vi "Controller_2_2_Proportional.vi"() -> ()   [LabVIEW 2019]
uses:
  <vilib>/myRIO/Instrument Drivers/Onboard IO/AI/typedefs/AI Reference.ctl
  <vilib>/myRIO/Common/Instrument Driver Framework/Utilities/typedefs/myRIO Generic Hardware Reference.ctl
  <vilib>/myRIO/Common/Instrument Driver Framework/Utilities/typedefs/Hardware Version Enum.ctl
  <vilib>/myRIO/Common/Instrument Driver Framework/Utilities/typedefs/myRIO v1.0 Reference.ctl
  <vilib>/myRIO/Common/Instrument Driver Framework/Utilities/typedefs/Generic FPGA Reference.ctl
  <vilib>/myRIO/Common/Instrument Driver Framework/myRIO v1.0/AI/typedefs/AI Channels List.ctl
  <vilib>/myRIO/Common/Instrument Driver Framework/myRIO v1.0/AI/typedefs/AI Channels Enum.ctl
  <vilib>/myRIO/Common/Instrument Driver Framework/Utilities/typedefs/Analog Scaling Constants List.ctl
  <vilib>/myRIO/Common/Instrument Driver Framework/Utilities/typedefs/Analog Scaling Constants.ctl
  <vilib>/userDefined/High Color/nirio_resource_hc.ctl
  <vilib>/Simulation/Scripting/Companion Diagram/SimConfigNode/SimParams.ctl
  <vilib>/Simulation/Scripting/Companion Diagram/SimConfigNode/_simSolvers.ctl
  <vilib>/Simulation/Implementation/Shared/SIMSCR Execution Mode.ctl
  <vilib>/Simulation/Param Hierarchy/Typedefs/SIMPH Param Control Actions.ctl
  <vilib>/myRIO/Instrument Drivers/Onboard IO/PWM/typedefs/PWM Reference.ctl
  <vilib>/myRIO/Common/Instrument Driver Framework/myRIO v1.0/PWM/typedefs/PWM Channels Enum.ctl
  <vilib>/myRIO/Instrument Drivers/Onboard IO/PWM/typedefs/PWM Configuration.ctl
  <vilib>/myRIO/Common/Instrument Driver Framework/Utilities/vis/Is FPGA Ref Available.vi
  <vilib>/myRIO/Common/Instrument Driver Framework/myRIO v1.0/AI/vis/myRIO v1.1 Open AI.vi
  <vilib>/myRIO/Instrument Drivers/Onboard IO/AI/vis/Read.vi
  <vilib>/Simulation/Implementation/Shared/NILVSim_ParamChanged.vi
  <vilib>/Simulation/Implementation/Shared/NILVSIM_BeginStep.vi
  <vilib>/Simulation/Implementation/Shared/NILVSim_Manager.vi
  <vilib>/Utility/error.llb/Clear Errors.vi
  <vilib>/Simulation/Implementation/Shared/NILVSim_FinalizeModel.vi
  <vilib>/myRIO/Common/Instrument Driver Framework/myRIO v1.0/PWM/vis/myRIO v1.1 Open PWM.vi
  <vilib>/myRIO/Instrument Drivers/Onboard IO/PWM/vis/Set Duty Cycle and Frequency.vi
  <vilib>/myRIO/Common/Instrument Driver Framework/Utilities/vis/Validate Channels.vi
  <vilib>/myRIO/Common/Instrument Driver Framework/myRIO v1.0/AI/vis/myRIO v1.0 Reserve AI.vi
  <vilib>/myRIO/Common/Instrument Driver Framework/myRIO v1.0/PWM/vis/myRIO v1.0 Reserve PWM.vi
  <vilib>/myRIO/Common/Instrument Driver Framework/myRIO v1.0/UART/vis/myRIO v1.0 Close UART.vi
  <vilib>/myRIO/Common/Instrument Driver Framework/myRIO v1.0/AI/vis/myRIO v1.0 Build MUX Configuration AI.vi
  <vilib>/myRIO/Common/Instrument Driver Framework/myRIO v1.0/Resource Manager/vis/myRIO v1.0 Reserve Channel List.vi
  <vilib>/myRIO/Common/Instrument Driver Framework/myRIO v1.0/PWM/vis/myRIO v1.0 Build MUX Configuration PWM.vi
  <vilib>/myRIO/Common/Instrument Driver Framework/myRIO v1.0/Resource Manager/vis/myRIO v1.0 Reserve Channel.vi
  <vilib>/myRIO/Common/Instrument Driver Framework/myRIO v1.0/Resource Manager/vis/myRIO v1.0 Unreserve Channel.vi
  <vilib>/myRIO/Common/Instrument Driver Framework/myRIO v1.0/Resource Manager/vis/myRIO v1.0 Create Configuration List.vi
  <vilib>/myRIO/Common/Instrument Driver Framework/myRIO v1.0/Resource Manager/vis/myRIO v1.0 Build Mutex Name.vi
  <vilib>/Utility/VariantDataType/GetNumericInfo.vi
  <vilib>/Utility/error.llb/Error Cluster From Error Code.vi
  <vilib>/myRIO/Common/Instrument Driver Framework/myRIO v1.0/myRIO v1.1 Open.vi
  <vilib>/myRIO/Common/Instrument Driver Framework/myRIO v1.0/AI/vis/myRIO v1.0 Get Scaling Constants AI.vi
  <vilib>/myRIO/Common/Instrument Driver Framework/Utilities/vis/IO Manager.vi
  <vilib>/myRIO/Common/Instrument Driver Framework/Utilities/vis/Configuration Manager.vi
  <vilib>/myRIO/Common/Instrument Driver Framework/myRIO v1.0/myRIO v1.0 Close.vi
  <vilib>/myRIO/Common/Instrument Driver Framework/myRIO v1.0/AI/vis/myRIO v1.0 Read AI.vi
  <vilib>/imath/engines/lvmath2/RunTimeEngine/Managers/WorkSpace/UID Generator.vi
  <vilib>/imath/engines/lvmath2/RunTimeEngine/RunTimeType/NIMS_RunTimeType_From StrictType (excl LVString).vi
  <instcachedir>/0/NIMS_RunTimeType_From StrictType (excl LVString)_D8AFBA86A94845AAA577C895450664BD.lvgen/NIMS_RunTimeType_From StrictType (excl LVString)_D8AFBA86A94845AAA577C895450664BD_000.vi
  <vilib>/imath/engines/lvmath2/RunTimeEngine/LocalVariableDefStatement/MC_LocalVariableDefStatement_Display.vi
  <vilib>/imath/engines/lvmath2/RunTimeEngine/Managers/SymbolTable/Clear UID.vi
  <vilib>/imath/engines/lvmath2/RunTimeEngine/NodeEndStatement/NIMS_NodeEndStatement_Output.vi
  <instcachedir>/0/NIMS_NodeEndStatement_Output_53EC0D466D134D7ABD903AC30B43404B.lvgen/NIMS_NodeEndStatement_Output_53EC0D466D134D7ABD903AC30B43404B_001.vi
  <vilib>/imath/engines/lvmath2/RunTimeEngine/ErrorHandling/NIMS_Finalize Error.vi
  <vilib>/Simulation/Implementation/Shared/SIM Unbundle Sim Info.vi
  <vilib>/Simulation/Implementation/Shared/NILVSim_Initialize.vi
  <vilib>/Simulation/Utility/Implementation/NILVSim Get Time and IsAcceptedStep.vi
  <vilib>/Simulation/Implementation/Shared/SIMSH Read Queue.vi
  <vilib>/Simulation/Implementation/Shared/NILVSim_GetModelError.vi
  <vilib>/Simulation/Implementation/Shared/SIM Bundle Sim Info.vi
  <vilib>/myRIO/Common/Instrument Driver Framework/myRIO v1.0/Resource Manager/vis/myRIO v1.0 Configure IO.vi
  <vilib>/myRIO/Common/Instrument Driver Framework/myRIO v1.0/PWM/vis/myRIO v1.0 Write PWM.vi
  <vilib>/addons/control/pid/pid.llb/PID (DBL).vi
  <vilib>/myRIO/Common/Instrument Driver Framework/Utilities/vis/FPGA Ref Manager.vi
  <vilib>/myRIO/Common/Instrument Driver Framework/myRIO v1.0/myRIO v1.0 Reset FPGA.vi
  <vilib>/myRIO/Common/Instrument Driver Framework/myRIO v1.0/IRQ/vis/myRIO v1.0 IRQ Info FGV.vi
  <vilib>/myRIO/Common/Instrument Driver Framework/myRIO v1.0/IRQ/vis/myRIO v1.0 Timer IRQ Info FGV.vi
  <vilib>/myRIO/Common/Instrument Driver Framework/myRIO v1.0/IRQ/vis/myRIO v1.0 ISR Agent.vi
  <vilib>/myRIO/Instrument Drivers/Utilities/vis/Reset Index.vi
  <vilib>/myRIO/Common/Instrument Driver Framework/myRIO v1.0/Resource Manager/vis/myRIO v1.0 Block Write Resource Manager.vi
  <vilib>/myRIO/Express VI/Onboard IO/AI/AI Express VI.xnode
  <vilib>/myRIO/Instrument Drivers/Onboard IO/AI/vis/myRIO AI Open.xnode
  <vilib>/Simulation/Implementation/XNodeFramework/SimXNode/SimX.xnode
  Subsystems/RateLimit.vi
  <vilib>/Simulation/Scripting/Companion Diagram/SimConfigNode/SimDog.xnode
  <vilib>/myRIO/Express VI/Onboard IO/PWM/PWM Express VI.xnode
  <vilib>/myRIO/Instrument Drivers/Onboard IO/PWM/vis/myRIO PWM Open.xnode
  <vilib>/myRIO/Instrument Drivers/Onboard IO/PWM/PWM.lvlib
  <vilib>/myRIO/Instrument Drivers/Onboard IO/AI/AI.lvlib
  <vilib>/imath/engines/lvmath2/RunTimeEngine/Managers/SymbolTable/NIMS_WorkSpace.lvlib
  <vilib>/addons/control/pid/NI_PID_pid.lvlib
  <vilib>/ptbypt/NI_PtbyPt.lvlib
  <vilib>/myRIO/Instrument Drivers/Utilities/Utilities.lvlib
  <vilib>/Simulation/Implementation/Shared/NI_SIM_Implementation.lvlib
panel:
  in  "emax 2":dbl
  in  "offset 2":dbl
  out "Duty Cycle 2":dynamicdata(graph)
  in  "emax":dbl
  in  "offset":dbl
  in  "Slew":dbl
  out "Deflate":dbl
  out "Inflate":dbl
  out "Deflate":bool
  out "Inflate":bool
  in  "deadband":dbl
  out "double precision float":dbl
  out "Arbitrary Signal":dynamicdata(graph)
  out "Duty Cycle":dynamicdata(graph)
  out "Pressure Actuator":dynamicdata(graph)
  out "Pressures Actuator":cluster{dbl, dbl}(knob)={0.0, 8.870406975580165} scale=0.0..120.0
  in  "stop":bool
  out "VA_sensor":dbl format="%#.3g"
  out "Pressures Receiver":cluster{dbl, dbl}(knob)={0.0, 8.870406975580165} scale=0.0..120.0
  in  "Setpoint Preceiver":dbl(slide) scale=0.0..100.0
  out "V_Rsensor":dbl format="%#.3g"
  in  "PID Motor":T1={"proportional gain (Kc)"=0.01, "integral time (Ti, min)"=0.005, "derivative time (Td, min)"=0.0} {"derivative time (Td, min)" format="%.3f"; "integral time (Ti, min)" format="%.3f"; "proportional gain (Kc)" format="%.3f"}
  out "Duty cycle Motor":dbl(knob) scale=0.0..1.0
  in  "milliseconds to wait":u32=100
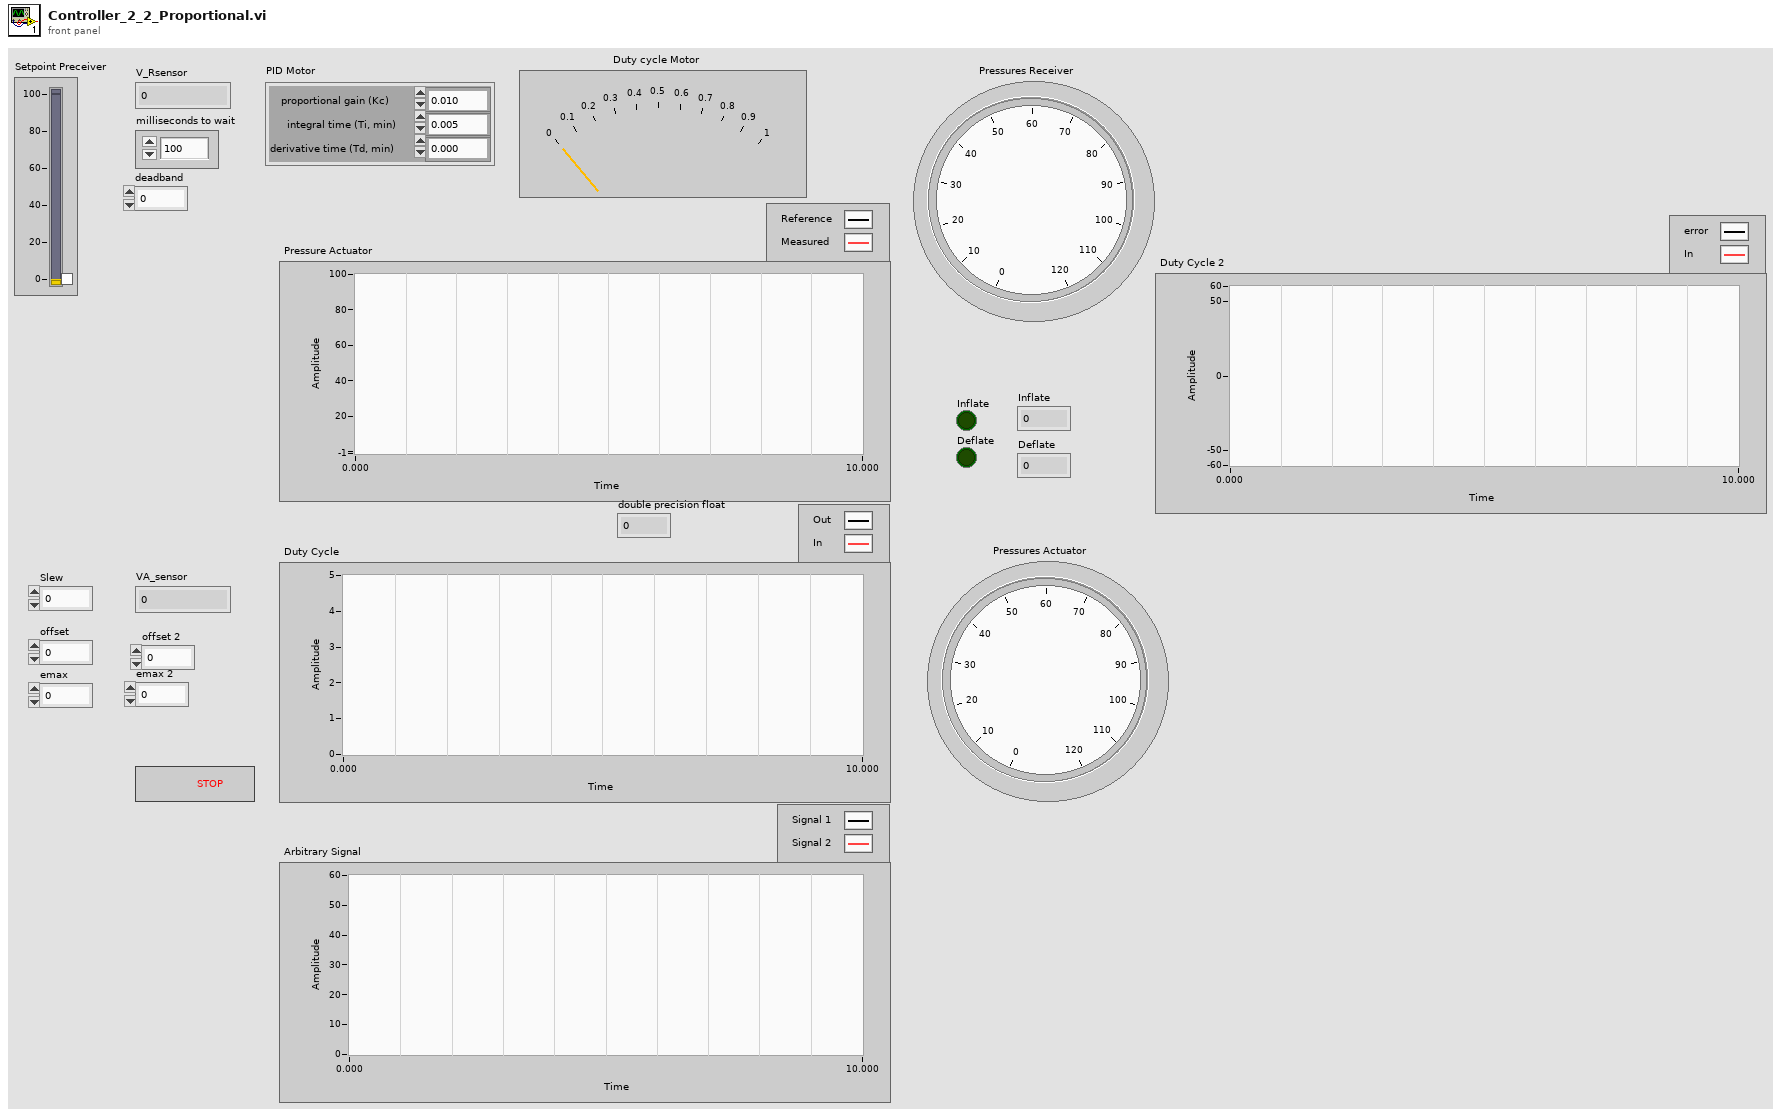
[diagram p1: front panel]
types:
  T1 = cluster{"proportional gain (Kc)":dbl, "integral time (Ti, min)":dbl, "derivative time (Td, min)":dbl}
  T2 = enum16{"Simulate to Completion", "Single Time-Step Simulation (Fixed Step Only)"}
  T3 = typedef "SIMSCR Execution Mode.ctl" = enum16{"Simulate to Completion", "Single Time-Step Simulation (Fixed Step Only)"}
  T4 = typedef "SIMPH Param Control Actions.ctl" = enum16{"get params", "set params"}
  T5 = cluster{"SIMSH Sim Time":dbl, "Negate":cluster{"-x":dbl}, "input":dbl, "Rate Limiter":cluster{"output":dbl}}
  T6 = typedef "SimParams.ctl" = cluster{"Initial Time (s)":dbl, "Final Time (s)":dbl, "Step Size (s)":dbl, "ODE Solver":T7, "Minimum Step Size (s)":dbl, "Maximum Step Size (s)":dbl, "Relative Tolerance":dbl, "Absolute Tolerance":dbl, "Software Timing":bool, "Initial Step Size (s)":dbl, "Automatic Fixed Step Size?":bool, "Automatic Discrete Step Size?":bool, "Discrete Step Size (s)":dbl, "Calculate using Time Step":bool, "Solver Wired?":bool, "Prev.Frm.Expected End":u64, "Prev.Frm.Actual End":u64, "Prev.Frm.Finished Late?":bool, "Prev.Iter.Expected End":u64, "Prev.Iter.Actual End":u64, "Prev.Iter.Finished Late?":bool, "Expected Iteration Start":u64, "Actual Iteration Start":u64, "Expected Frame Start":u64, "Actual Frame Start":u64, "Source Name":string, "Name":string, "Period":i64, "Deadline":i64, "Offset":i64, "Start":i64, "Priority":i32, "Timeout":i32, "Processor":i32, "Mode":enum32{"No Change", "Process missed periods, maintain original phase", "Discard missed periods, maintain original phase", "Process missed periods, ignore original phase", "Discard missed periods, ignore original phase"}, "Wakeup reason":enum32{"Normal", "Aborted", "Asynchronous wakeup", "Timing source error", "Timed loop error", "Timeout"}, "Error":errorcluster, "Source Type":string, "Secondary Source Type":string, "Global End Time":u64, "Global Start Time":u64, "Full Solver Reset":bool, "Execution Mode":T3, "Nan/Inf Check":bool, "Custom Solver Library":string, "Solver Is Variable":bool, "custom solver name":string, "Signal Collection Decimation":u32}
  T7 = typedef "_simSolvers.ctl" = enum16{"Runge-Kutta 1 (Euler)", "Runge-Kutta 2", "Runge-Kutta 3", "Runge-Kutta 4", "Runge-Kutta 23 (variable)", "Runge-Kutta 45 (variable)", "BDF (variable)", "Adams-Moulton (variable)", "Rosenbrock (variable)", "Discrete States Only", "SDIRK 4 (variable)", "Radau 5 (variable)", "Radau 9 (variable)", "Radau 13 (variable)", "Radau [Variable Order] (variable)", "Gear's Method (variable)", "Linearizer", "State Query", "Trim Eval", "Custom Solver"}
  T8 = typedef "PWM.lvlib/PWM Reference.ctl" = cluster{"myRIO Reference":T9, "PWM Channels Enum":T13, "PWM Configuration":T14}
  T9 = typedef "myRIO Generic Hardware Reference.ctl" = cluster{"myRIO Model":T10, "myRIO Hardware Reference":T11}
  T10 = typedef "Hardware Version Enum.ctl" = enum16{"Unknown", "myRIO-1900", "myRIO-1950", "roboRIO", "NI ELVIS RIO CM", "ELVIS III"}
  T11 = typedef "myRIO v1.0 Reference.ctl" = cluster{"Generic FPGA Reference":T12, "Allow multiple opens":bool}
  T12 = typedef "Generic FPGA Reference.ctl" = refnum<k20>
  T13 = typedef "PWM Channels Enum.ctl" = enum16{"Not Connected", "C/PWM0", "C/PWM1", "A/PWM0", "A/PWM1", "A/PWM2", "A/PWM3", "A/PWM4", "A/PWM5", "A/PWM6", "A/PWM7", "A/PWM8", "A/PWM9", "A/PWM10", "A/PWM11", "A/PWM12", "A/PWM13", "A/PWM14", "A/PWM15", "A/PWM16", "A/PWM17", "A/PWM18", "A/PWM19", "B/PWM0", "B/PWM1", "B/PWM2", "B/PWM3", "B/PWM4", "B/PWM5", "B/PWM6", "B/PWM7", "B/PWM8", "B/PWM9", "B/PWM10", "B/PWM11", "B/PWM12", "B/PWM13", "B/PWM14", "B/PWM15", "B/PWM16", "B/PWM17", "B/PWM18", "B/PWM19", "PWM/PWM0", "PWM/PWM1", "PWM/PWM2", "PWM/PWM3", "PWM/PWM4", "PWM/PWM5", "PWM/PWM6", "PWM/PWM7", "PWM/PWM8", "PWM/PWM9"}
  T14 = typedef "PWM.lvlib/PWM Configuration.ctl" = cluster{"Frequency":dbl, "Duty Cycle":dbl}
  T15 = typedef "nirio_resource_hc.ctl" = tag
  T16 = typedef "AI.lvlib/AI Reference.ctl" = cluster{"myRIO Reference":T9, "AI Channels List":T17, "AI Scaling Constants List":T19}
  T17 = typedef "AI Channels List.ctl" = T18[]
  T18 = typedef "AI Channels Enum.ctl" = enum16{"Not Connected", "AudioIn/Left", "AudioIn/Right", "C/AI0", "C/AI1", "A/AI0", "A/AI1", "A/AI2", "A/AI3", "A/AI4", "A/AI5", "A/AI6", "A/AI7", "B/AI0", "B/AI1", "B/AI2", "B/AI3", "B/AI4", "B/AI5", "B/AI6", "B/AI7", "AI/AI0", "AI/AI1", "AI/AI2", "AI/AI3", "A/AI0 (DIFF)", "A/AI1 (DIFF)", "A/AI2 (DIFF)", "A/AI3 (DIFF)", "B/AI0 (DIFF)", "B/AI1 (DIFF)", "B/AI2 (DIFF)", "B/AI3 (DIFF)"}
  T19 = typedef "Analog Scaling Constants List.ctl" = T20[]
  T20 = typedef "Analog Scaling Constants.ctl" = cluster{"LSB Weight (Volts)":dbl, "Offset (Volts)":dbl, "Signed?":bool}
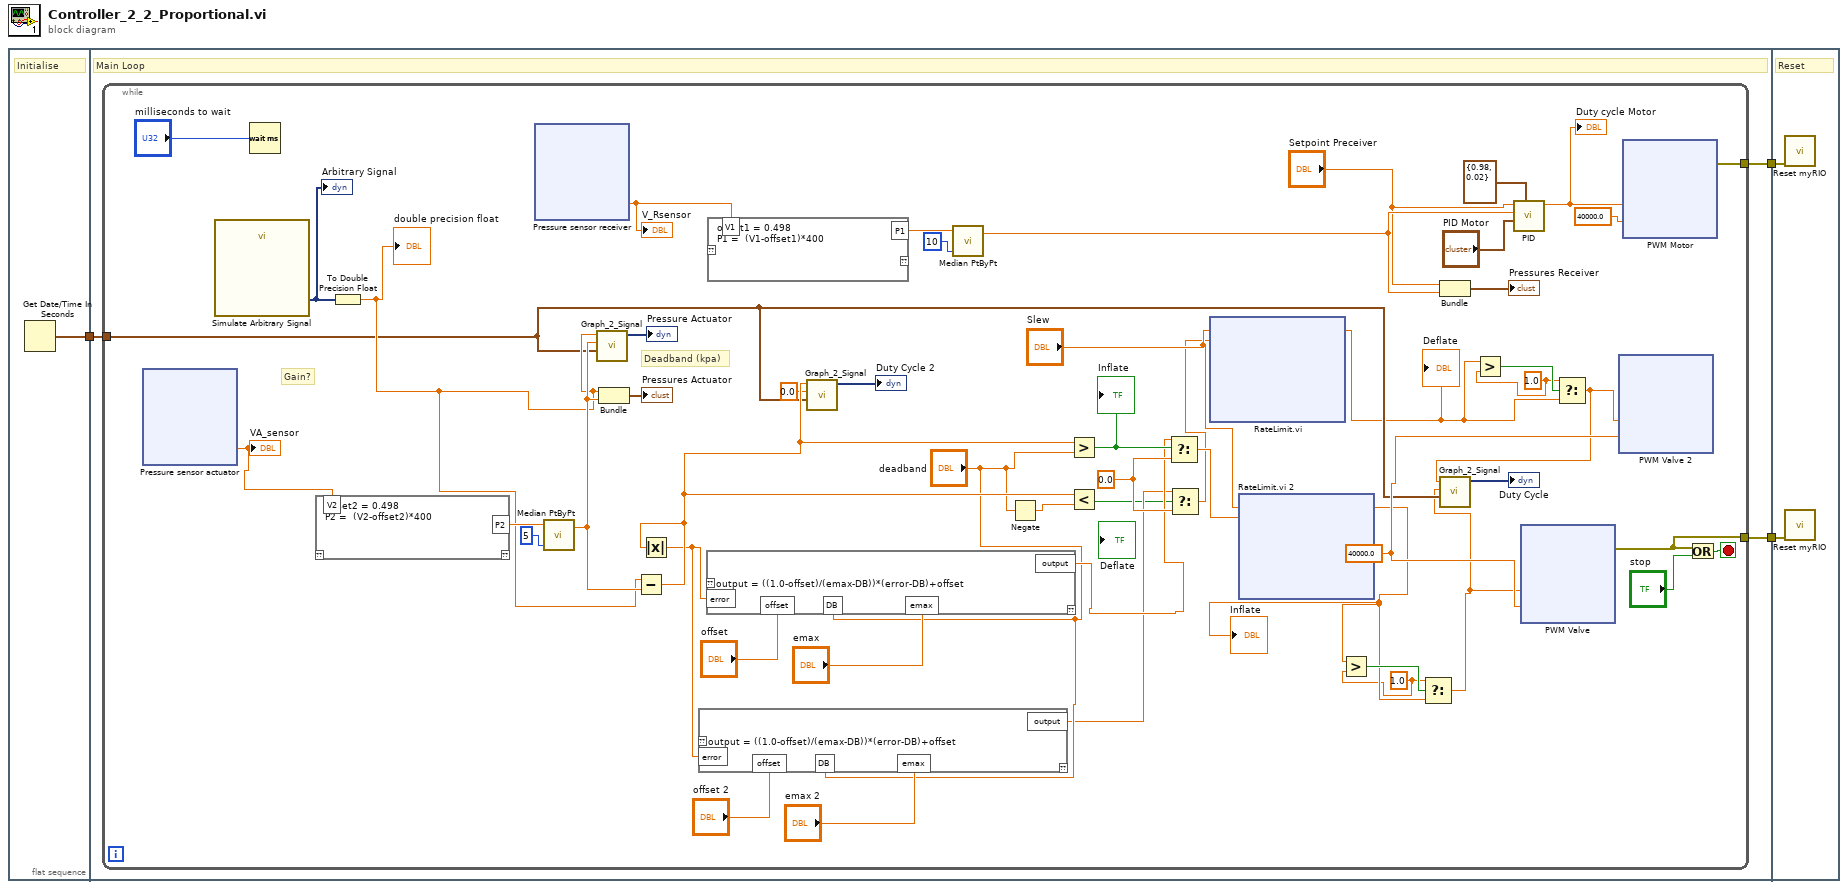
[diagram p0: block diagram]
diagram:
  n1 = flat-sequence {
    tunnel: [w4] -> w3
    tunnel: [w7] -> w2
    tunnel: [w6] -> w1
    tunnel: w3 -> [w5]
    tunnel: w2 -> [w938]
    tunnel: w1 -> [w937]
    frame #0 {
      # "Initialise"
      n2 = Get Date/Time In Seconds() -> (seconds since 1Jan1904=w4:timestamp)
    }
    frame #1 {
      # "Main Loop"
      n3 = while {
        tunnel: [w58] -> w7
        tunnel: [w47] -> w6
        tunnel: w5 -> [w23]
        stop <- w57 stop-if-true
        w11 = 1.0 ("t")
        w13 = 1.0 ("t")
        w34 = 0.0 ("f")
        w37 = 40000.0 ("Frequency [Hz]")
        # "Deadband (kpa)"
        # "Gain?"
        n4 = xnode "Pressure sensor actuator"() -> ("B/AI1 (Pin 5)"=w42:dbl)  [unwired: 1 in, 1 out]
        "VA_sensor" <- w42
        n5 = call "Simulate Arbitrary Signal"() -> ("Signal"=w40:dynamicdata)  [unwired: 9 in, 2 out]
        "Arbitrary Signal" <- w40
        n6 = Wait (ms)(milliseconds to wait="milliseconds to wait") -> ()  [unwired: 1 out]
        n7 = mathscript code="offset2 = 0.498\nP2 =  (V2-offset2)*400"("V2"=w42) -> ("P2"=w56:dbl)  [unwired: 1 in, 1 out]
        n8 = To Double Precision Float(number=w40) -> (double precision float=w27:dbl)
        "double precision float" <- w27
        n9 = xnode "Pressure sensor receiver"() -> ("B/AI0 (Pin 3)"=w41:dbl)  [unwired: 1 in, 1 out]
        "V_Rsensor" <- w41
        n10 = call <vilib>:"Median PtByPt.vi"("sample length"=5, "x"=w56) -> ("median"=w36:dbl)  [unwired: 2 in, 1 out]
        n11 = call "Graph_2_Signal.vi"("y"=w23, "Dynamic Data 2"=w36, "Dynamic Data 1"=w27) -> ("Signals"=→"Pressure Actuator":dynamicdata)  [unwired: 8 in]
        n12 = Bundle(w27, "median"=w36) -> (→"Pressures Actuator":cluster{dbl, "median":dbl})  [unwired: 1 in]
        n13 = Subtract(x=w27, y=w36) -> (x-y=w24:dbl)
        n14 = Absolute Value(x=w24) -> (abs(x)=w19:dbl)
        n15 = mathscript code="output = ((1.0-offset)/(emax-DB))*(error-DB)+offset"("error"=w19, "offset"="offset 2", "DB"="deadband", "emax"="emax 2") -> ("output"=w17:dbl)  [unwired: 1 in, 1 out]
        n16 = mathscript code="output = ((1.0-offset)/(emax-DB))*(error-DB)+offset"("error"=w19, "offset"="offset", "DB"="deadband", "emax"="emax") -> ("output"=w26:dbl)  [unwired: 1 in, 1 out]
        n17 = mathscript code="offset1 = 0.498\nP1 =  (V1-offset1)*400"("V1"=w41) -> ("P1"=w49:dbl)  [unwired: 1 in, 1 out]
        n18 = call "Graph_2_Signal.vi"("y"=w23, "Dynamic Data 2"=0.0, "Dynamic Data 1"=w24) -> ("Signals"=→"Duty Cycle 2":dynamicdata)  [unwired: 8 in]
        n19 = call <vilib>:"Median PtByPt.vi"("sample length"=10, "x"=w49) -> ("median"=w51:dbl)  [unwired: 2 in, 1 out]
        n20 = Negate(x="deadband") -> (-x=w33:dbl)
        n21 = Greater?(x=w24, y="deadband") -> (0:w35:bool)
        "Inflate" <- w35
        n22 = Less?(x=w24, y=w33) -> (x < y?=w16:bool)
        n23 = Select(t=w26, s=w35, f=w34) -> (s? t:f=w32:dbl)
        n24 = Select(t=w17, s=w16, f=w34) -> (s? t:f=w30:dbl)
        n25 = xnode "RateLimit.vi"("slew rate"="Slew", "input"=w30) -> ("output"=w10:dbl)  [unwired: 2 in, 10 out]
        "Deflate" <- w10
        n26 = xnode "RateLimit.vi 2"("slew rate"="Slew", "input"=w32) -> ("output"=w14:dbl)  [unwired: 2 in, 10 out]
        "Inflate" <- w14
        n27 = Greater?(x=w14, y=w13) -> (0:w15:bool)
        n28 = Select(t=w13, s=w15, f=w14) -> (s? t:f=w8:dbl)
        n29 = Bundle("Setpoint Preceiver"="Setpoint Preceiver", "median"=w51) -> (→"Pressures Receiver":cluster{"Setpoint Preceiver":dbl, "median":dbl})  [unwired: 1 in]
        n30 = Greater?(x=w10, y=w11) -> (0:w12:bool)
        n31 = call-poly <vilib>:"PID.vi"("output range"=cluster{"output high":dbl, "output low":dbl} {"output high"=0.98, "output low"=0.02} ("output range motor"), "PID gains"="PID Motor", "process variable"=w51, "setpoint"="Setpoint Preceiver") -> ("output"=w38:dbl)  [unwired: 6 in, 1 out]
        "Duty cycle Motor" <- w38
        n32 = xnode "PWM Valve"("Duty Cycle"=w8, "Frequency [Hz]"=w37) -> ("error out"=w58:errorcluster)  [unwired: 1 in]
        n33 = Select(t=w11, s=w12, f=w10) -> (s? t:f=w9:dbl)
        n34 = call "Graph_2_Signal.vi"("y"=w23, "Dynamic Data 2"=w8, "Dynamic Data 1"=w9) -> ("Signals"=→"Duty Cycle":dynamicdata)  [unwired: 8 in]
        n35 = xnode "PWM Valve 2"("Duty Cycle"=w9, "Frequency [Hz]"=w37) -> ()  [unwired: 1 in, 1 out]
        n36 = xnode "PWM Motor"("Duty Cycle"=w38, "Frequency [Hz]"=40000.0) -> ("error out"=w47:errorcluster)  [unwired: 1 in]
        n37 = Or(x=w58, y="stop") -> (x .or. y?=w57:bool)
      }
    }
    frame #2 {
      # "Reset"
      n38 = call <vilib>:"Reset myRIO.vi"("error in (no error)"=w937) -> ()  [unwired: 10 in, 1 out]
      n39 = call <vilib>:"Reset myRIO.vi"("error in (no error)"=w938) -> ()  [unwired: 10 in, 1 out]
    }
  }
